vi "Z900_navX_Util_EncodeProtocol_SignedHundredths.vi"(1 "Signed Hundredths (0.00)":dbl[](array[numeric])) -> (0 "Little Endian":u8[](array[numeric]))   [LabVIEW 2016, in "navX Library.lvlib"]
uses:
  navX Library.lvlib
  Z900_navX_Util_BigEndian_to_LittleEndian.vi
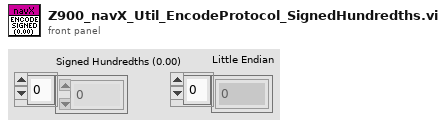
[diagram p1: front panel]
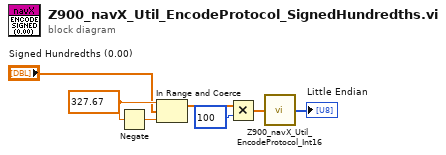
[diagram p0: block diagram]
diagram:
  w4 = 327.67
  n1 = Negate(x=w4) -> (-x=w3:dbl)
  n2 = In Range and Coerce(upper limit=w4, x="Signed Hundredths (0.00)", lower limit=w3) -> (coerced(x)=w1:dbl[])  [unwired: 1 out]
  n3 = Multiply(x=w1, y=100) -> (x*y=w6:dbl[])
  n4 = call "Z900_navX_Util_EncodeProtocol_Int16.vi"("Int16"=w6) -> ("Little Endian"=→"Little Endian":u8[])
